vi "Self Alias.vi"(11 "Base jettl in":refnum<class "Base jettl.lvclass">) -> (2 "Self Alias":string)   [LabVIEW 2021, in "jettl.lvlib" / "Base jettl.lvclass"]
uses:
  Base jettl.lvclass
  Base jettl.lvclass/Base jettl.ctl
  Addresses Strategy/Addresses Strategy/Addresses Strategy.lvclass
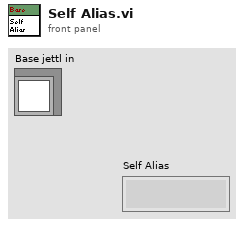
[diagram p1: front panel]
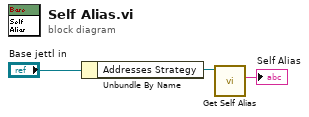
[diagram p0: block diagram]
diagram:
  n1 = Unbundle By Name("Base jettl in") -> ("Addresses Strategy"=w3:refnum<class "Addresses Strategy.lvclass">)
  n2 = call-dynamic "Get Self Alias.vi"("Addresses Strategy in"=w3) -> ("Self Alias"=→"Self Alias":string)  [unwired: 10 in]
